vi "登陆界面.vi"() -> ()   [LabVIEW 2011]
panel:
  in  "停止":bool
  # "用户登陆系统"
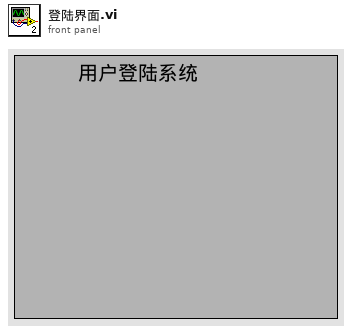
[diagram p1: front panel]
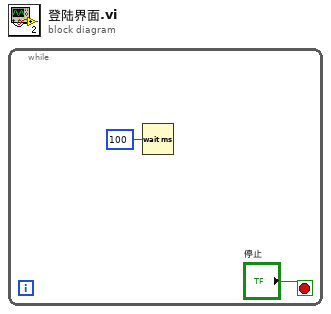
[diagram p0: block diagram]
diagram:
  n1 = while {
    stop <- "停止" stop-if-true
    n2 = Wait (ms)(milliseconds to wait=u32 100 ("等待时间（毫秒）")) -> ()  [unwired: 1 out]
  }
